vi "Get MetaData from Results.vi"(8 "error in":errorcluster, 10 "measurement plugin service in":refnum<class "Measurement Plugin Service.lvclass">, 11 "results cluster":variant) -> (0 "error out":errorcluster, 2 "measurement plugin service out":refnum<class "Measurement Plugin Service.lvclass">, 3 "outputs":T1[](array[typedef]))   [LabVIEW 2021, in "NI Measurement Plug-In SDK.lvlib"]
uses:
  NI Measurement Plug-In SDK.lvlib
  TypeDefs/Output Parameter.ctl
  TypeDefs/Parameter Annotations Entry.ctl
  Measurement Plugin Service/Measurement Plugin Service.lvclass
  <vilib>/Utility/Data Type/NI_Data Type.lvlib
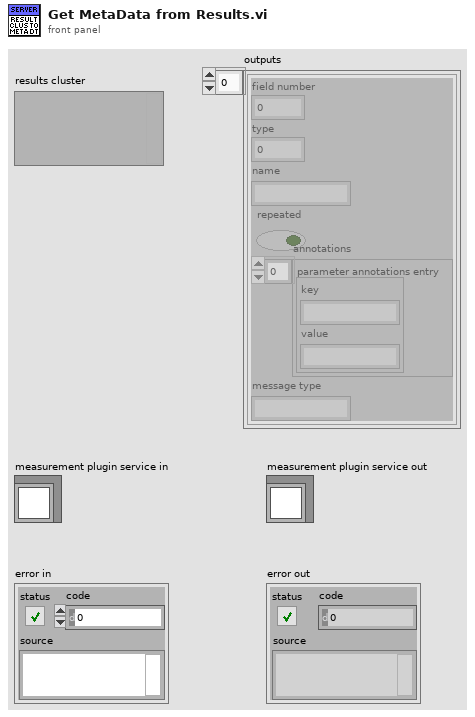
[diagram p1: front panel]
types:
  T1 = typedef "NI Measurement Plug-In SDK.lvlib/Output Parameter.ctl" = cluster{"field number":i32, "type":i32, "name":string, "repeated":bool, "annotations":T2[], "message type":string}
  T2 = typedef "NI Measurement Plug-In SDK.lvlib/Parameter Annotations Entry.ctl" = cluster{"key":string, "value":string}
  T3 = typedef "NI Measurement Plug-In SDK.lvlib/Measurement Plugin Service.lvclass/Plugin Paths.ctl" = cluster{"get service descriptor VI path":path, "get type specializations VI path":path, "get UI details VI path":path, "measurement logic VI path":path, "measurement configuration ctl path":path, "measurement results ctl path":path}
  T4 = cluster{"Parameter Name":string, "Annotations":T2[]}[]
  T5 = typedef "NI Measurement Plug-In SDK.lvlib/Google Protobuf Field Kind.ctl" = enum32{"TYPE_UNKNOWN", "TYPE_DOUBLE", "TYPE_FLOAT", "TYPE_INT64", "TYPE_UINT64", "TYPE_INT32", "TYPE_FIXED64", "TYPE_FIXED32", "TYPE_BOOL", "TYPE_STRING", "TYPE_GROUP", "TYPE_MESSAGE", "TYPE_BYTES", "TYPE_UINT32", "TYPE_ENUM", "TYPE_SFIXED32", "TYPE_SFIXED64", "TYPE_SINT32", "TYPE_SINT64"}
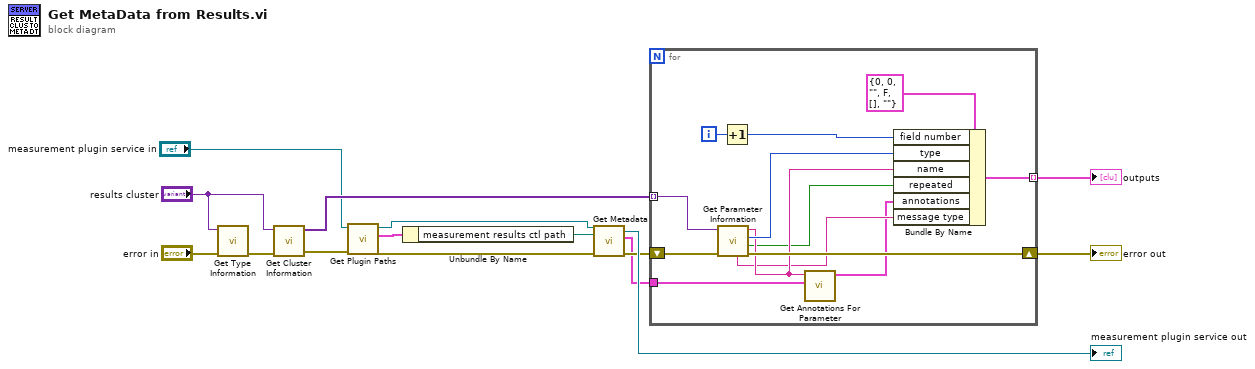
[diagram p0: block diagram]
diagram:
  n1 = call <vilib>:"Get Type Information.vi"("error in (no error)"="error in", "variant"="results cluster") -> ("error out"=w15:errorcluster)  [unwired: 5 in, 4 out]
  n2 = call <vilib>:"Get Cluster Information.vi"("error in (no error)"=w15, "variant"="results cluster") -> ("error out"=w4:errorcluster, "cluster elements"=w14:variant[])  [unwired: 8 in]
  n3 = call-dynamic "Get Plugin Paths.vi"("error in"=w4, "measurement plugin service in"="measurement plugin service in") -> ("error out"=w7:errorcluster, "plugin paths"=w11:T3, "measurement plugin service out"=w3:refnum<class "Measurement Plugin Service.lvclass">)  [unwired: 7 in]
  n4 = Unbundle By Name(w11) -> ("measurement results ctl path"=w10:path)
  n5 = call "Get Metadata.vi"("error in"=w7, "measurement control path"=w10, "measurement plugin service in"=w3) -> ("error out"=w8:errorcluster, "metadata value"=w5:T4, "measurement plugin service out"=→"measurement plugin service out":refnum<class "Measurement Plugin Service.lvclass">)  [unwired: 5 in]
  n6 = for {
    tunnel: w14 -> [w26] mode=indexing
    shift-right: [w24] -> w2
    shift-left: w8 -> [w25]
    tunnel: w5 -> [w27]
    tunnel: [w22] -> w1 mode=indexing
    i -> [w28]
    n7 = call "Get Parameter Information.vi"("error in"=w25, "variant data"=w26) -> ("error out"=w24:errorcluster, "repeated"=w18:bool, "grpc type"=w20:T5, "name"=w19:string, "message type"=w17:string)  [unwired: 5 in]
    n8 = Increment(x=w28) -> (x+1=w21:i32)
    n9 = call "Get Annotations For Parameter.vi"("metadata value"=w27, "parameter name"=w19) -> ("annotations"=w16:T2[])  [unwired: 9 in]
    n10 = Bundle By Name(cluster=T1 {"field number"=0, "type"=0, "name"="", "repeated"=FALSE, "annotations"=[], "message type"=""} ("OutputParameter"), "field number"=w21, "type"=w20, "name"=w19, "repeated"=w18, "annotations"=w16, "message type"=w17) -> (w22:T1)
  }
  "error out" <- w2
  "outputs" <- w1
